vi "UpdateChnlDelaysHW.vi"(8 "error in (no error)":errorcluster, 11 "BME_DG_Base in":refnum<class "BME_DG_Base.lvclass">) -> (0 "error out":errorcluster, 3 "BME_DG_Base out":refnum<class "BME_DG_Base.lvclass">)   [LabVIEW 2009, in "POLARIS BME DG.lvlib" / "BME_DG_Base.lvclass"]
doc: "Currently just a Wrapper for SetChannelHW.vi. In future may realise channeling pattern with preprocessing (e.g. Deactivate) and postprocessing (e.g. Activate) operations around SetChannelHW.\n\nauthor: Alexander Kessler, Helmholtz-Institut-Jena \nmaintainer: Alexander Kessler: alexander.kessler@uni-jena.de\n\nLast Change:\nLicense Agreement for this software:\n\nCopyright (C)\nHelmholtz-Institut-Jena\nFröbelsteg 3\n07743 Jena\nGermany\n\nContact: alexander.kessler@uni-jena.de\n\nThis program is free software; you can redistribute it and/or modify it under the terms of the GNU General Public License as published by the Free Software Foundation; either version 2 of the license, or (at your option) any later version.\n\nThis program is distributed in the hope that it will be useful, but WITHOUT ANY WARRANTY; without even the implied warranty of MERCHANTABILITY or FITNESS FOR A PARTICULAR PURPOSE. See the GNU General License for more details (http://www.gnu.org)."
uses:
  BME_DG_Base.lvclass
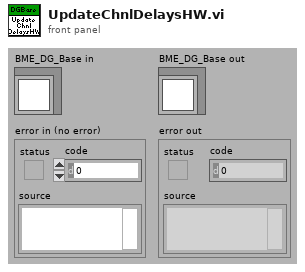
[diagram p1: front panel]
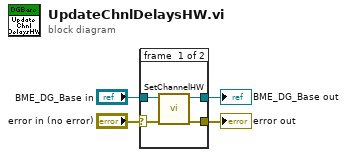
[diagram p0: block diagram]
diagram:
  n1 = case shown="No Error" "error in (no error)" {
    selector: "error in (no error)" -> [w6 w10]
    tunnel: [w5 w10] -> w3
    tunnel: [w7 w9] -> w1
    tunnel: "BME_DG_Base in" -> [w8 w9]
    frame #0 {
      n2 = call-dynamic "SetChannelHW.vi"("error in (no error)"=w6, "BME_DG_Base in"=w8) -> ("error out"=w5:errorcluster, "BME_DG_Base out"=w7:refnum<class "BME_DG_Base.lvclass">)  [unwired: 8 in]
    }
    frame #1 {
    }
  }
  "error out" <- w3
  "BME_DG_Base out" <- w1
